vi "GetItemArray.vi"(8 "Error":errorcluster, 11 "Tree in":refnum<class "Tree.lvclass">) -> (0 "Error":errorcluster, 1 "TopVisible":string, 2 "TreeItems[]":T1(array[cluster]), 3 "Tree out":refnum<class "Tree.lvclass">)   [LabVIEW 2021, in "Tree.lvlib" / "Tree.lvclass"]
uses:
  Tree.lvclass
  Tree.lvclass/Tree.ctl
  Private/TreeControllerTag.ctl
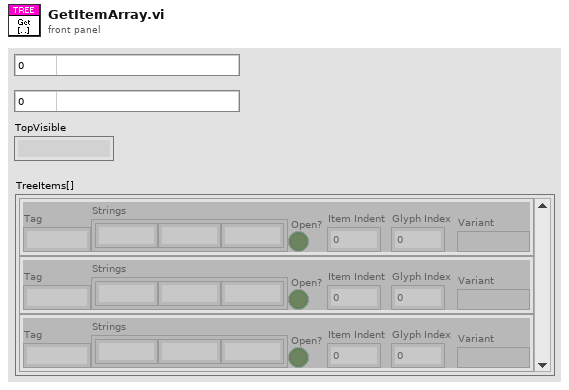
[diagram p1: front panel]
types:
  T1 = cluster{"Tag":string, "Strings":string[], "Open?":bool, "Item Indent":i32, "Glyph Index":i32, "Variant":variant}[]
  T2 = typedef "Tree.lvlib/Tree.lvclass/TreeControllerTag.ctl" = enum8{"Null", "1. Add item", "2. Delete item", "3. Get All Tree Data", "4. Drag Starting", "5. Drag Ended", "6. Add Tree Values", "7. Get Item Value", "8. Edit Item", "9. StepBack", "10. Filter"}
  T3 = cluster{"Node":string, cluster{"Tag":string, "Strings":string[], "Open?":bool, "Item Indent":i32, "Glyph Index":i32, "Variant":variant}[]}
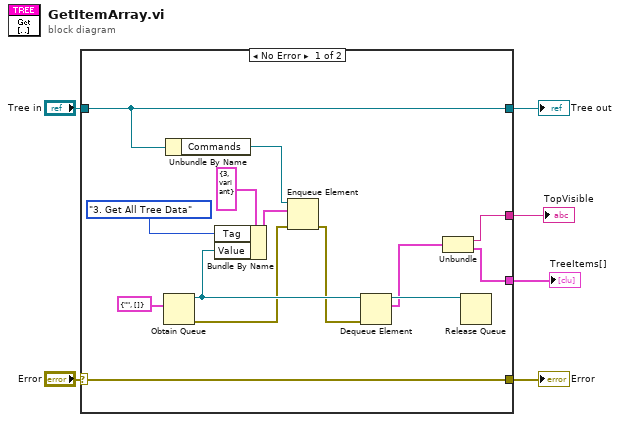
[diagram p0: block diagram]
diagram:
  n1 = case shown="No Error" "Error" {
    selector: "Error" -> [w20 w22]
    tunnel: [w20 w22] -> w5
    tunnel: [w19 w21] -> w3
    tunnel: "Tree in" -> [w19 w21]
    tunnel: [w9 _] -> w2
    tunnel: [w8 _] -> w1
    frame No Error {
      n2 = Obtain Queue(element data type=T3 {"Node"="", []} ("output cluster")) -> (queue out=w16:refnum<queue>, error out=w13:errorcluster)  [unwired: 4 in, 1 out]
      n3 = Unbundle By Name(w19) -> ("Commands"=w12:refnum<queue>)
      n4 = Bundle By Name(cluster=cluster{"Tag":u8, "Value":variant} {"Tag"=3, "Value"=variant} ("element"), "Tag"=TreeControllerTag."3. Get All Tree Data", "Value"=w16) -> (w17:cluster{"Tag":u8, "Value":variant})
      n5 = Enqueue Element(queue=w12, element=w17, error in (no error)=w13) -> (error out=w14:errorcluster)  [unwired: 1 in, 2 out]
      n6 = Dequeue Element(queue=w16, error in (no error)=w14) -> (queue out=w15:refnum<queue>, element=w10:T3)  [unwired: 1 in, 2 out]
      n7 = Unbundle(w10) -> ("Node"=w9:string, w8:T1)
      n8 = Release Queue(queue=w15) -> ()  [unwired: 2 in, 3 out]
    }
    frame Error {
    }
  }
  "Error" <- w5
  "Tree out" <- w3
  "TopVisible" <- w2
  "TreeItems[]" <- w1
